vi "Append Block To Response.vi"(11 "Block Upload Sub-Block Transfer in":refnum<class "Block Upload Sub-Block Transfer.lvclass">) -> (3 "Block Upload Sub-Block Transfer out":refnum<class "Block Upload Sub-Block Transfer.lvclass">)   [LabVIEW 2020, in "CANopen.lvlib" / "SDO Manager.lvlib" / "Block Upload Sub-Block Transfer.lvclass"]
uses:
  Block Upload Sub-Block Transfer.lvclass
  D:/git/CANopen-LabVIEW/source/SDO Manager/SDO Manager/SDO Transfer/SDO Transfer.lvclass
  SDO Transfer/SDO Transfer.lvclass/SDO Transfer.ctl
  Block Upload Sub-Block Transfer.lvclass/Block Upload Sub-Block Transfer.ctl
  SDO Transfer/SDO Transfer.lvclass
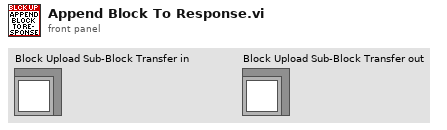
[diagram p1: front panel]
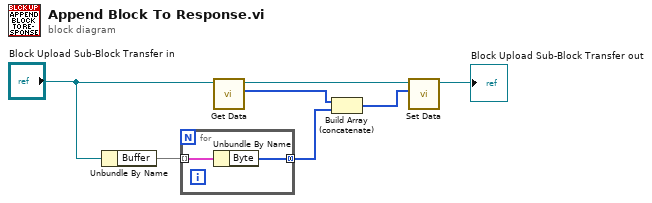
[diagram p0: block diagram]
diagram:
  n1 = Unbundle By Name("Block Upload Sub-Block Transfer in") -> ("Buffer"=w5:map{u8, u8[]})
  n2 = for {
    tunnel: [w8] -> w2 mode=concatenating
    tunnel: w5 -> [w9] mode=indexing
    n3 = Unbundle By Name(w9) -> ("Byte"=w8:u8[])
  }
  n4 = call "Get Data.vi"("SDO Transfer in"="Block Upload Sub-Block Transfer in") -> ("Data"=w3:u8[], "SDO Transfer out"=w4:refnum<class "Block Upload Sub-Block Transfer.lvclass">)  [unwired: 8 in, 1 out]
  n5 = Build Array (concatenate)(w3, w2) -> (w1:u8[])
  n6 = call "Set Data.vi"("Data"=w1, "SDO Transfer in"=w4) -> ("SDO Transfer out"=→"Block Upload Sub-Block Transfer out":refnum<class "Block Upload Sub-Block Transfer.lvclass">)  [unwired: 8 in, 1 out]
